vi "HVBuncher.CalculateVoltage.vi"(10 "nomVoltages":dbl[](array[numeric])) -> (2 "ChannelVoltages":dbl[](array[numeric]))   [LabVIEW 2014, in "HVBuncher.lvlib"]
uses:
  HVBuncher.lvlib
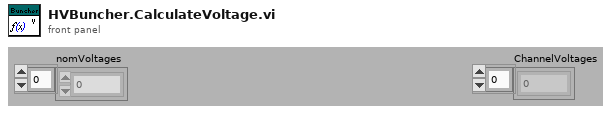
[diagram p1: front panel]
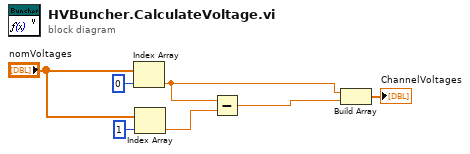
[diagram p0: block diagram]
diagram:
  n1 = Index Array(array="nomVoltages", index=0) -> (element=w3:dbl)
  n2 = Index Array(array="nomVoltages", index=1) -> (element=w4:dbl)
  n3 = Subtract(x=w3, y=w4) -> (x-y=w2:dbl)
  n4 = Build Array(w3, w2) -> (→"ChannelVoltages":dbl[])
